vi "listen.vi"(6 "timeout ms (10000)":i32=10000, 8 "error in":errorcluster, 11 "Queue server in":refnum<class "Queue server.lvclass">) -> (0 "error out":errorcluster, 1 "valid?":bool, 2 "new connection":refnum<class "connection maintainer.lvclass">, 3 "Queue server out":refnum<class "Queue server.lvclass">, 5 "client ID":string)   [LabVIEW 2015, in "Queue server.lvclass"]
uses:
  Queue server.lvclass
  connection/connection maintainer.lvclass
  Queue server.lvclass/Queue server.ctl
  Queue connection/Queue connection.lvclass
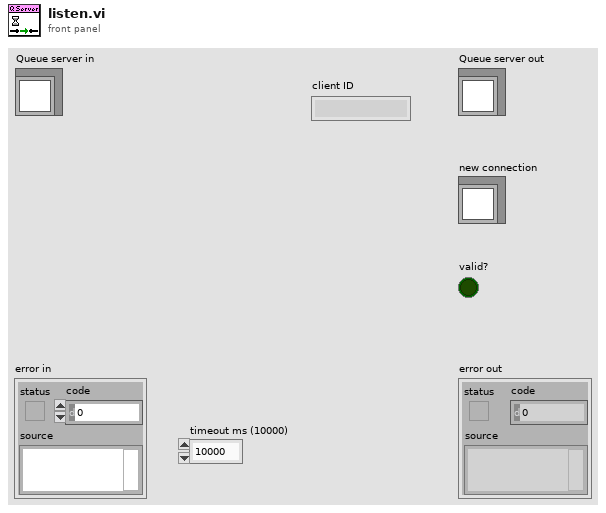
[diagram p1: front panel]
types:
  T1 = typedef "Queue connection.lvclass/queue pair.ctl" = cluster{"to pair":refnum<queue>, "from pair":refnum<queue>}
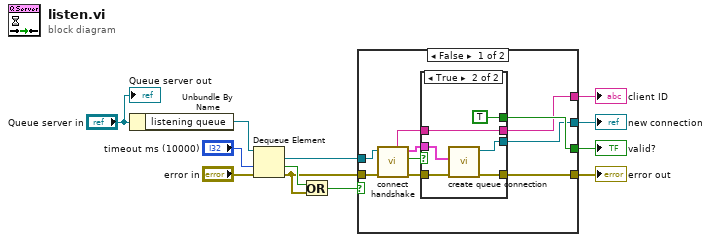
[diagram p0: block diagram]
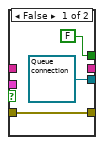
[diagram p2: hidden frame]
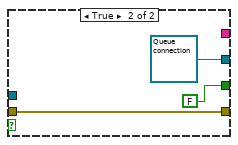
[diagram p3: hidden frame]
diagram:
  n1 = Unbundle By Name("Queue server in") -> ("listening queue"=w6:refnum<queue>)
  n2 = Dequeue Element(queue=w6, timeout in ms (-1)="timeout ms (10000)", error in (no error)="error in") -> (element=w12:refnum<class "communicator message.lvclass">, timed out?=w10:bool, error out=w9:errorcluster)  [unwired: 1 out]
  n3 = Or(x=w10, y=w9) -> (x .or. y?=w11:bool)
  n4 = case shown="False" w11 {
    tunnel: w12 -> [w22 _]
    tunnel: w9 -> [w18 w34]
    tunnel: [w17 w34] -> w4
    tunnel: [w16 FALSE] -> w3
    tunnel: [w15 refnum<class "Queue connection.lvclass"> refnum ("TCP connection out")] -> w2
    tunnel: [w14 _] -> w1
    frame False {
      n5 = call "connect handshake.vi"("error in"=w18, "message"=w22) -> ("error out"=w21:errorcluster, "valid?"=w19:bool, "queues"=w20:T1, "client ID"=w13:string)  [unwired: 6 in]
      n6 = case shown="True" w19 {
        tunnel: w21 -> [w25 w31]
        tunnel: w20 -> [_ w30]
        tunnel: [w25 w29] -> w17
        tunnel: [FALSE TRUE] -> w16
        tunnel: [refnum<class "Queue connection.lvclass"> refnum ("TCP connection out") w27] -> w15
        tunnel: [_ w26] -> w14
        tunnel: w13 -> [_ w26]
        frame False {
        }
        frame True {
          n7 = call "create queue connection.vi"("error in"=w31, "queues"=w30) -> ("error out"=w29:errorcluster, "TCP connection out"=w27:refnum<class "Queue connection.lvclass">)  [unwired: 8 in]
        }
      }
    }
    frame True {
    }
  }
  "error out" <- w4
  "new connection" <- w2
  "valid?" <- w3
  "client ID" <- w1
  "Queue server out" <- "Queue server in"
